vi "get_process_layer_parameters_cluster.vi"(8 "error in (no error)":errorcluster, 9 "Layer number":u8, 10 "Process number":u8, 11 "VISA resource name":refnum<visa-resource-name>) -> (0 "error out":errorcluster, 2 "Process layer parameters":T1, 3 "VISA resource name out":refnum<visa-resource-name>)   [LabVIEW 2018]
doc: "Set the density of a material."
uses:
  Low Level/process_layer_parameter_ring.ctl
  Low Level/process_layer_parameters_strings.ctl
  Low Level/process_layer_parameters.ctl
panel:
  in  "Process layer parameters (strings)":T2
  in  "Process layer parameter":T3 items=["Material", "Final Thick (kA)", "Thick Limit (kA)", "Crucible", "CoDep", "Ratio Cntrl (%)"]
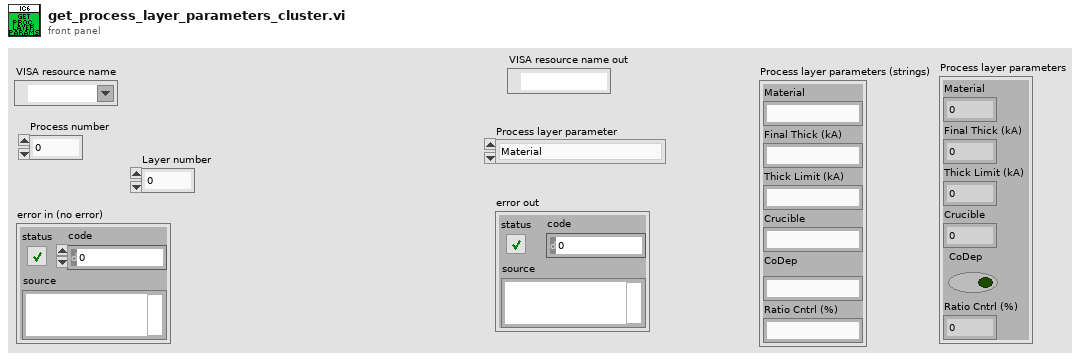
[diagram p1: front panel]
types:
  T1 = typedef "process_layer_parameters.ctl" = cluster{"Material":u8, "Final Thick (kA)":sgl, "Thick Limit (kA)":sgl, "Crucible":u8, "CoDep":bool, "Ratio Cntrl (%)":sgl}
  T2 = typedef "process_layer_parameters_strings.ctl" = cluster{"Material":string, "Final Thick (kA)":string, "Thick Limit (kA)":string, "Crucible":string, "CoDep":string, "Ratio Cntrl (%)":string}
  T3 = typedef "process_layer_parameter_ring.ctl" = u16
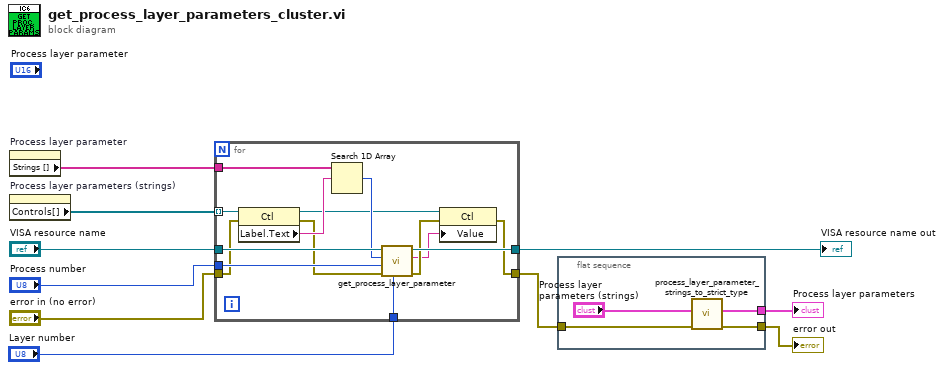
[diagram p0: block diagram]
diagram:
  n1 = property on="Process layer parameter" class="Ring (strict)"() -> ("Strings []"=w6:string[])  [unwired: 2 in, 2 out]
  n2 = property on="Process layer parameters (strings)" class="Clust (strict)"() -> ("Controls[]"=w5:refnum<vi>[])  [unwired: 2 in, 2 out]
  n3 = for {
    tunnel: "VISA resource name" -> [w24]
    tunnel: [w23] -> w9
    tunnel: [w12] -> w3
    tunnel: "error in (no error)" -> [w17]
    tunnel: "Process number" -> [w22]
    tunnel: w6 -> [w21]
    tunnel: w5 -> [w20] mode=indexing
    tunnel: "Layer number" -> [w11]
    n4 = property class="Ctl"(reference=w20, error in=w17) -> (reference out=w15:refnum<vi>, error out=w16:errorcluster, "Label.Text"=w19:string)
    n5 = Search 1D Array(1D array=w21, element=w19) -> (index of element=w18:i32)  [unwired: 1 in]
    n6 = call "get_process_layer_parameter.vi"("Layer number"=w11, "error in (no error)"=w16, "Process number"=w22, "Process layer parameter"=w18, "VISA resource name"=w24) -> ("error out"=w14:errorcluster, "Process layer parameter value"=w13:string, "VISA resource name out"=w23:refnum<visa-resource-name>)  [unwired: 4 in]
    n7 = property class="Ctl"(reference=w15, error in=w14, "Value"=w13) -> (error out=w12:errorcluster)  [unwired: 1 out]
  }
  "VISA resource name out" <- w9
  n8 = flat-sequence {
    tunnel: [w26] -> w4
    tunnel: w3 -> [w27]
    tunnel: [w25] -> w2
    frame #0 {
      n9 = call "process_layer_parameter_strings_to_strict_type.vi"("error in (no error)"=w27, "Process layer parameters (strings)"="Process layer parameters (strings)") -> ("error out"=w26:errorcluster, "Process layer parameters"=w25:T1)  [unwired: 8 in]
    }
  }
  "error out" <- w4
  "Process layer parameters" <- w2
